vi "Skip current RUN.vi"(8 "error in (no error)":errorcluster, 11 "Run Block in":refnum<class "Run Block.lvclass">) -> (0 "error out":errorcluster, 3 "Run Block out":refnum<class "Run Block.lvclass">)   [LabVIEW 2020, in "TALOS.lvlib" / "Run Utilities.lvlib" / "Run Block.lvclass"]
doc: "Adds Current RUN to Skipped RUNs. If Reinstert is true, it throws it at the top of the skipped list"
uses:
  Run Block.lvclass
  Schedule/Schedule.lvclass
  Run Instance/Run Instance.lvclass
  Run Block.lvclass/Run Block.ctl
  Cell/Schedule Cell.lvclass
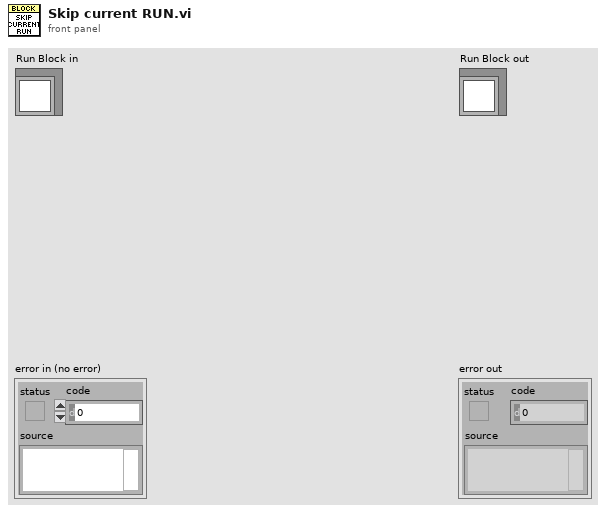
[diagram p1: front panel]
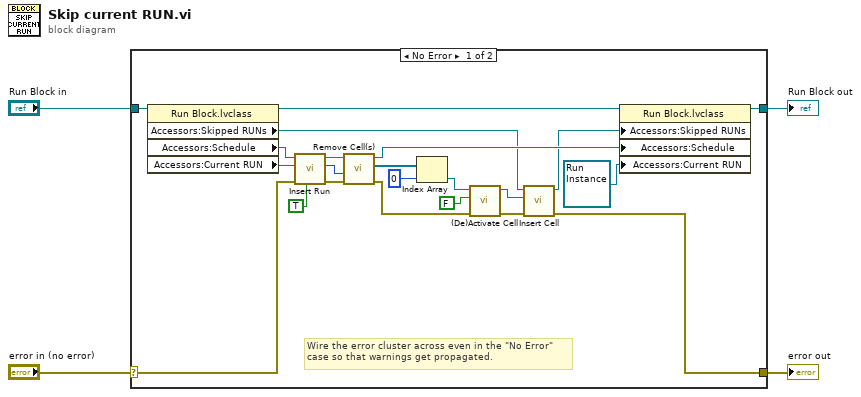
[diagram p0: block diagram]
diagram:
  n1 = case shown="No Error" "error in (no error)" {
    selector: "error in (no error)" -> [w26 w28]
    tunnel: [w8 w28] -> w3
    tunnel: [w24 w27] -> w1
    tunnel: "Run Block in" -> [w25 w27]
    frame No Error {
      # "Wire the error cluster across even in the \"No Error\"\ncase so that warnings get propagated."
      n2 = property class="Run Block.lvclass"(reference=w25) -> (reference out=w23:refnum<class "Run Block.lvclass">, "Accessors:Skipped RUNs"=w10:refnum<class "Schedule.lvclass">, "Accessors:Schedule"=w21:refnum<class "Schedule.lvclass">, "Accessors:Current RUN"=w22:refnum<class "Run Instance.lvclass">)  [unwired: 1 in, 1 out]
      n3 = call-dynamic "Insert Run.vi"("Reinsert?"=TRUE, "error in (no error)"=w26, "Run Instance"=w22, "Schedule in"=w21) -> ("error out"=w18:errorcluster, "Index"=w19:i32, "Schedule out"=w20:refnum<class "Schedule.lvclass">)  [unwired: 5 in]
      n4 = call-dynamic "Remove Cell(s).vi"("error in (no error)"=w18, "index"=w19, "Schedule in"=w20) -> ("error out"=w12:errorcluster, "Deleted Cell(s)"=w16:refnum<class "Schedule Cell.lvclass">[], "Schedule out"=w17:refnum<class "Schedule.lvclass">)  [unwired: 6 in]
      n5 = Index Array(array=w16, index=0) -> (element=w13:refnum<class "Schedule Cell.lvclass">)
      n6 = call-dynamic "(De)Activate Cell.vi"("error in (no error)"=w12, "Active"=FALSE, "Schedule Cell in"=w13) -> ("error out"=w7:errorcluster, "Schedule Cell out"=w6:refnum<class "Schedule Cell.lvclass">)  [unwired: 7 in]
      n7 = call-dynamic "Insert Cell.vi"("error in (no error)"=w7, "Schedule Cell"=w6, "Schedule in"=w10) -> ("error out"=w8:errorcluster, "Schedule out"=w9:refnum<class "Schedule.lvclass">)  [unwired: 7 in]
      n8 = property class="Run Block.lvclass"(reference=w23, "Accessors:Skipped RUNs"=w9, "Accessors:Schedule"=w17, "Accessors:Current RUN"=refnum<class "Run Instance.lvclass"> refnum ("Current RUN")) -> (reference out=w24:refnum<class "Run Block.lvclass">)  [unwired: 1 in, 1 out]
    }
    frame Error {
    }
  }
  "error out" <- w3
  "Run Block out" <- w1
